vi "PH_SM_Class.constructor.vi"(0 "name":string, 2 "data in":string, 5 "error in":errorcluster) -> (14 "i ref out":refnum<vi>, 16 "data out":string, 19 "error out":errorcluster)   [LabVIEW 2014, in "PH_SM_Class.lvlib"]
doc: "This class is forseen to be inherited from. With its help data of devices can be stored in the PHELIX shot data base (PSDB). \n\n\n\nauthor: Stefan Götte, GSI\n\nLicense Agreement for this software:\n\nCopyright (C)\nGesellschaft für Schwerionenforschung, GSI\nPlanckstr. 1\n64291 Darmstadt\nGermany\n\nContact: D.Beck@gsi.de \n\nThis program is free software; you can redistribute it and/or modify it under the terms of the \nGNU General Public License as published by the Free Software Foundation; either version 2 of \nthe license, or (at your option) any later version.\n\nThis program is distributed in the hope that it will be useful, but WITHOUT ANY WARRANTY; \nwithout even the implied warranty of MERCHANTABILITY or FITNESS FOR A PARTICULAR PURPOSE. See the GNU General License for more details (http://www.gnu.org).\n\nGesellschaft für Schwerionenforschung, GSI\nPlanckstr. 1, 64291 Darmstadt, Germany\nFor all questions and ideas contact: M.Richter@gsi.de, H.Brand@gsi.de or D.Beck@gsi.de.\nLast update: 16-JUN-2004"
uses:
  PH_SM_Class.lvlib
  CS_Core/CSSystem/CSSystemLib/CSSystemLib.lvlib
  CS_Core/BaseProcess/BaseProcess.lvlib
  CS_Core/BaseSM/BaseSM.lvlib
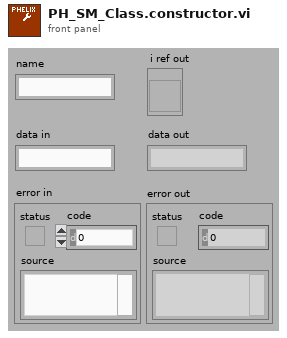
[diagram p1: front panel]
types:
  T1 = typedef "BaseProcess.lvlib/BaseProcess.i attribute.ctl" = cluster{"EventStatus":string, "EventError":i32, "PresetEvtWatchD":i32, "PresetPdcWatchD":i32, "EventTimeout":i32, "PeriodicInterval":i32, "Interface":string[], "Address":string[], "Special":string[], "PeriodicError":i32, "PeriodicStatus":string, "SuperProc":string, "Descriptors":T2[], "CaseRef":refnum<vi>, "PdcRef":refnum<vi>, "Thread Ref":refnum<vi>, "eventErrorID":i32, "eventStatusID":i32, "periodicErrorID":i32, "periodicStatusID":i32, "pdcCtrID":i32}
  T2 = typedef "BaseProcess.lvlib/BaseProcess.descriptor definition.ctl" = cluster{"selector":string, "descriptor":T3}
  T3 = typedef "BaseProcess.lvlib/BaseProcess.descriptor string definition.ctl" = string
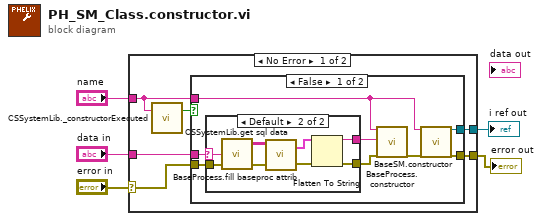
[diagram p0: block diagram]
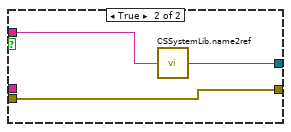
[diagram p3: hidden frame]
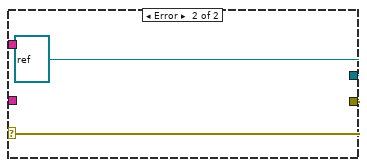
[diagram p4: hidden frame]
diagram:
  n1 = case shown="No Error" "error in" {
    selector: "error in" -> [w11 w34]
    tunnel: [w8 refnum<vi> refnum ("i ref out")] -> w5
    tunnel: [w9 w34] -> w4
    tunnel: "name" -> [w7 _]
    tunnel: "data in" -> [w10 _]
    frame No Error {
      n2 = call "CSSystemLib._constructorExecuted.vi"("name"=w7) -> ("constructor executed?"=w6:bool)  [unwired: 18 in]
      n3 = case shown="False" w6 {
        tunnel: w11 -> [w19 w30]
        tunnel: w10 -> [w17 _]
        tunnel: w7 -> [w16 w32]
        tunnel: [w13 w30] -> w9
        tunnel: [w12 w31] -> w8
        frame False {
          n4 = case shown="Default" w17 {
            selector: w17 -> [w20 w22]
            tunnel: w19 -> [w21 w27]
            tunnel: [w21 w25] -> w15
            tunnel: [w20 w23] -> w18
            frame "", "N/A" {
            }
            frame Default {
              n5 = call "CSSystemLib.get sql data.vi"("error in (no error)"=w27, "object"=w22) -> ("error out"=w29:errorcluster, "queryResults"=w28:string[][])  [unwired: 1 in, 1 out]
              n6 = call "BaseProcess.fill baseproc attrib.vi"("error in (no error)"=w29, "queryResults"=w28) -> ("error out"=w26:errorcluster, "cluster out"=w24:T1)  [unwired: 1 in]
              n7 = Flatten To String(anything=w24, error in (no error)=w26) -> (data string=w23:string, error out=w25:errorcluster)  [unwired: 2 in, 1 out]
            }
          }
          n8 = call "BaseProcess.constructor.vi"("name"=w16, "data in"=w18, "error in (no error)"=w15) -> ("error out"=w14:errorcluster)  [unwired: 14 in, 2 out]
          n9 = call "BaseSM.constructor.vi"("name"=w16, "error in (no error)"=w14) -> ("i ref out"=w12:refnum<vi>, "error out"=w13:errorcluster)  [unwired: 15 in, 1 out]
        }
        frame True {
          n10 = call "CSSystemLib.name2ref.vi"("name"=w32) -> ("obj refnum"=w31:refnum<vi>)
        }
      }
    }
    frame Error {
    }
  }
  "i ref out" <- w5
  "error out" <- w4
